vi "DFT.vi"(1 "Input":cdb[](array[numeric])) -> (0 "Output":cdb[](array[numeric]))   [LabVIEW 2018]
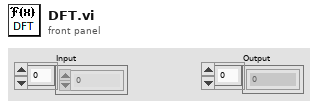
[diagram p1: front panel]
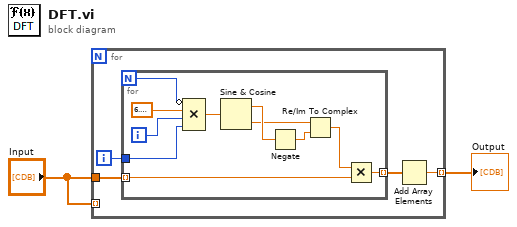
[diagram p0: block diagram]
diagram:
  n1 = for {
    tunnel: [w4] -> w2 mode=indexing
    tunnel: "Input" -> [w3]
    tunnel: "Input" -> [_] mode=indexing
    i -> [w6]
    n2 = for {
      N -> [w16]
      tunnel: [w12] -> w5 mode=indexing
      tunnel: w6 -> [w14]
      tunnel: w3 -> [w13] mode=indexing
      i -> [w15]
      n3 = Compound Arithmetic op=MULTIPLY(invert w16, 6.283185307179586, w15, w14) -> (w9:dbl)
      n4 = Sine & Cosine(0:w9) -> (1:w8:dbl, 2:w7:dbl)
      n5 = Negate(x=w8) -> (-x=w11:dbl)
      n6 = Re/Im To Complex(1:w11, 2:w7) -> (0:w10:cdb)
      n7 = Multiply(x=w10, y=w13) -> (x*y=w12:cdb)
    }
    n8 = Add Array Elements(numeric array=w5) -> (sum=w4:cdb)
  }
  "Output" <- w2
